vi "Status SpecimenTempCtrlSettings(SCP).vi"(8 "error in (no error)":errorcluster, 10 "Address (0)":i32, 11 "VISA resource name":refnum<visa-resource-name>) -> (0 "error out":errorcluster, 1 "Temp. Data":T1, 2 "control permission/state":bool, 3 "VISA resource name out":refnum<visa-resource-name>, 4 "lower deviation":dbl, 5 "upper deviation":dbl)   [LabVIEW 2016, in "Environment Chamber.lvlib" / "Climatic Chamber.lvlib"]
doc: "<b>Operating specimen temperature control monitor</B>\n\nReturns the specimen temperature control state."
uses:
  Climatic Chamber.lvlib
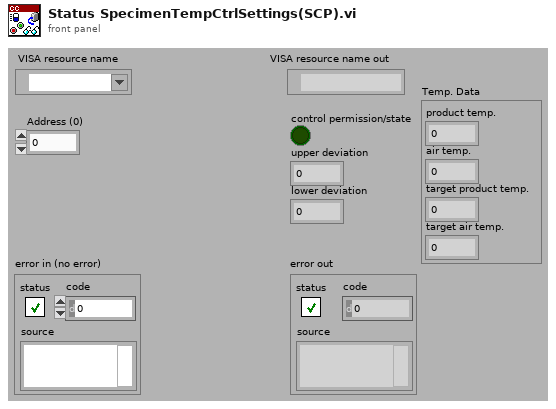
[diagram p1: front panel]
types:
  T1 = cluster{"product temp.":dbl, "air temp.":dbl, "target product temp.":dbl, "target air temp.":dbl}
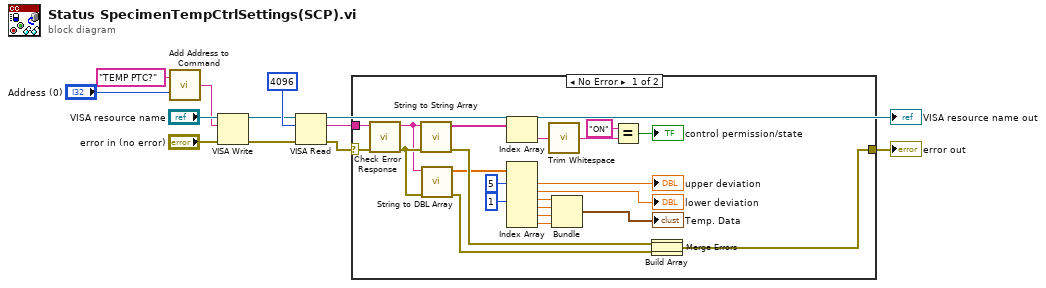
[diagram p0: block diagram]
diagram:
  n1 = call "Add Address to Command.vi"("Address (0)"="Address (0)", "Command"="TEMP PTC?") -> ("Command OUT"=w5:string)
  n2 = VISA Write(VISA resource name="VISA resource name", write buffer=w5, error in (no error)="error in (no error)") -> (VISA resource name out=w9:refnum<visa-resource-name>, error out=w8:errorcluster)  [unwired: 1 out]
  n3 = VISA Read(VISA resource name=w9, byte count=u32 4096, error in (no error)=w8) -> (VISA resource name out=→"VISA resource name out":refnum<visa-resource-name>, read buffer=w3:string, error out=w4:errorcluster)  [unwired: 1 out]
  n4 = case shown="No Error" w4 {
    selector: w4 -> [w33 w36]
    tunnel: w3 -> [w34 _]
    tunnel: [w19 w36] -> w2
    frame No Error {
      n5 = call "Check Error Response.vi"("error in (no error)"=w33, "read String"=w34) -> ("error out"=w27:errorcluster, "String out"=w26:string)  [unwired: 7 in, 1 out]
      n6 = call "String to String Array.vi"("error in (no error)"=w27, "String received"=w26) -> ("error out"=w35:errorcluster, "Array Data"=w32:string[])  [unwired: 8 in]
      n7 = call "String to DBL Array.vi"("error in (no error)"=w27, "String received"=w26) -> ("error out"=w20:errorcluster, "Array Data"=w25:dbl[])  [unwired: 8 in]
      n8 = Index Array(array=w32) -> (element=w31:string)  [unwired: 1 in]
      n9 = Index Array(array=w25, index #1=5 ("index"), index #3=1 ("index")) -> (element #1=→"upper deviation":dbl, element #2=→"lower deviation":dbl, element #3=w18:dbl, element #4=w17:dbl, element #5=w16:dbl, element #6=w15:dbl)  [unwired: 4 in]
      n10 = call <vilib>:"Trim Whitespace.vi"("string"=w31) -> ("trimmed string"=w30:string)  [unwired: 1 in]
      n11 = Bundle(w18, w17, w16, w15) -> (→"Temp. Data":cluster{dbl, dbl, dbl, dbl})  [unwired: 1 in]
      n12 = Equal?(x="ON", y=w30) -> (x = y?=→"control permission/state":bool)
      n13 = Build Array(w35, w20) -> (w13:errorcluster[])
      n14 = Merge Errors(w13) -> (w19:errorcluster)
    }
    frame Error {
    }
  }
  "error out" <- w2
